vi "crio_FPGA_VCA_Force_Sine_Sweep.vi"() -> ()   [LabVIEW 2019]
uses:
  <vilib>/LabVIEW Targets/FPGA/cRIO/shared/nicrio_ModuleControls/nicrio_cRIO-9237_ExcitationVoltageRing.ctl
  <vilib>/LabVIEW Targets/FPGA/cRIO/shared/nicrio_ModuleControls/nicrio_cRIO-9237_DataRatesRing.ctl
  <vilib>/Platform/TimedLoop/XDataNode/timing_clust.ctl
  <vilib>/Platform/TimedLoop/XDataNode/nitl_modes.ctl
  <vilib>/Platform/TimedLoop/XDataNode/wakeup.ctl
  <vilib>/rvi/FXPMathLib/basic elements/FxpIntAccumulator/subVIs/nifxpmath_IntAccumulator_SimConfig.ctl
  <vilib>/rvi/FXPMathLib/FxpRectToPolar/subVIs/nifxpmath_RectToPolar_SimConfig.ctl
  <vilib>/rvi/Emulation/niFpgaSctlEmulationGetInTimedLoop.vi
  <vilib>/rvi/Emulation/niFpgaProcessEmulError.vi
  <vilib>/rvi/eio/common/nirviEmuTemplateMethod_errors.vi
  <vilib>/rvi/eio/common/nirviEmuTemplatePropertySet_errors.vi
  <vilib>/rvi/Emulation/niFpgaGetClockAttributes.vi
  <vilib>/rvi/Emulation/niFpgaEmulationReportErrorSimple.vi
  <vilib>/rvi/Emulation/niFpgaCriticalErrorInLSC.vi
  <vilib>/rvi/Analysis/common/codeGenErrors/XNode/niFpgaXNodeCodeGenErrorHandle.vi
  <vilib>/rvi/FXPMathLib/basic elements/FxpIntAccumulator/simVIs/DllFxpIntAccumulator_sub.vi
  <vilib>/rvi/FXPMathLib/FxpRectToPolar/simVIs/DllFxpRectToPolarTemp_sub.vi
  <vilib>/eio/EIOMethodNode/EIOMethodNode.xnode
  <vilib>/eio/EIOPropertyNode/EIOPropertyNode.xnode
  <vilib>/eio/EIONode/EIONode.xnode
  <vilib>/rvi/FXPMathLib/FxpInterpret/XNode/nifxpmath_Interpret.xnode
  <vilib>/rvi/FXPMathLib/FxpMul/XNode/nifxpmath_Multiplier.xnode
  <vilib>/rvi/FXPMathLib/FxpAdd/XNode/nifxpmath_Add.xnode
  <vilib>/rvi/Analysis/measure/mean-var-std/XNode/niFpgaMean-Var-Std.xnode
  <vilib>/platform/TimedLoop/XDataNode/XDataNode.xnode
  <vilib>/rvi/FXPMathLib/basic elements/FxpIntAccumulator/XNode/nifxpmath_IntAccumulator.xnode
  <vilib>/rvi/FXPMathLib/FxpRectToPolar/XNode/nifxpmath_RectToPolar.xnode
  <vilib>/rvi/FXPMathLib/sim/FxpSim.dll
  <vilib>/Platform/TimedLoop/XDataNode/XDNodeRunTimeDep.lvlib
  <vilib>/rvi/eio/common/nirviEmuTemplatePropertyGet_errors.vi
  <vilib>/rvi/eio/common/nirviEmuTemplatePropertyGet_noerrors.vi
  <vilib>/rvi/eio/common/nirviEmuTemplatePropertySet_noerrors.vi
panel:
  out "scaled load cell reading":fxp<+/-,24,24>
  out "error out":errorcluster {"code" format="%.0x"}
  in  "Data Rate":T1=1 items=["50.000 kS/s (NI 9237)"=1, "25.000 kS/s (NI 9237)"=2, "16.667 kS/s (NI 9237)"=3, "12.500 kS/s (NI 9237)"=4, "10.000 kS/s (NI 9237)"=5, "8.333 kS/s (NI 9237)"=6, "7.143 kS/s (NI 9237)"=7, "6.250 kS/s (NI 9237)"=8, "5.556 kS/s (NI 9237)"=9, "5.000 kS/s (NI 9237)"=10, "4.545 kS/s (NI 9237)"=11, "4.167 kS/s (NI 9237)"=12, "3.846 kS/s (NI 9237)"=13, "3.571 kS/s (NI 9237)"=14, "3.333 kS/s (NI 9237)"=15, "3.125 kS/s (NI 9237)"=16, "2.941 kS/s (NI 9237)"=17, "2.778 kS/s (NI 9237)"=18, "2.632 kS/s (NI 9237)"=19, "2.500 kS/s (NI 9237)"=20, "2.381 kS/s (NI 9237)"=21, "2.273 kS/s (NI 9237)"=22, "2.174 kS/s (NI 9237)"=23, "2.083 kS/s (NI 9237)"=24, "2.000 kS/s (NI 9237)"=25, "1.923 kS/s (NI 9237)"=26, "1.852 kS/s (NI 9237)"=27, "1.786 kS/s (NI 9237)"=28, "1.724 kS/s (NI 9237)"=29, "1.667 kS/s (NI 9237)"=30, "1.613 kS/s (NI 9237)"=31]
  in  "Excitation Voltage":T2 items=["2.5 Volts", "3.3 Volts", "5.0 Volts", "10.0 Volts", "External Excitation"]
  in  "Half-Bridge Enable":bool
  in  "Finite?":bool=TRUE
  in  "Samples per Channel":u32=1000
  out "Mod1/AI0":fxp<+/-,24,-4>
  in  "Loop Rate (uSec)":u32
  in  "Shunt Cal Enable":bool
  in  "sweep frequency (periods/tick)":fxp<+,32,0>=1.25030055642128e-06
  out "sine out":i16
  out "sin_fxp":fxp<+/-,16,1>
  out "cos_fxp":fxp<+/-,16,1>
  out "cosine out":i16
  in  "Lock_loop_rate":u32 caption="Count(uSec)"
  in  "Lock_debug":bool
  out "magnitude":fxp<+,32,6>
  out "phase (pi)":fxp<+/-,16,2>
  out "output valid":bool
  out "sin*input":fxp<+/-,32,6>
  out "cos*input":fxp<+/-,32,6>
  out "lock_input":fxp<+/-,24,24>
  in  "sin_gain":fxp<+,32,1>=0.5
  in  "sin_offset":fxp<+/-,16,3>=0.5
  out "ControllerPWM Output":sgl
  in  "stop":bool
  in  "DC PWM Period (microsec)":i16=50
  # "1Hz -> sweep frequency: 2.5e-8\n5H -> 1.25e-7"
  # "DRV8256 Specs:\n\n0 0: Brake Low\n1 1: Brake High\nPWM 0\n0 PWM"
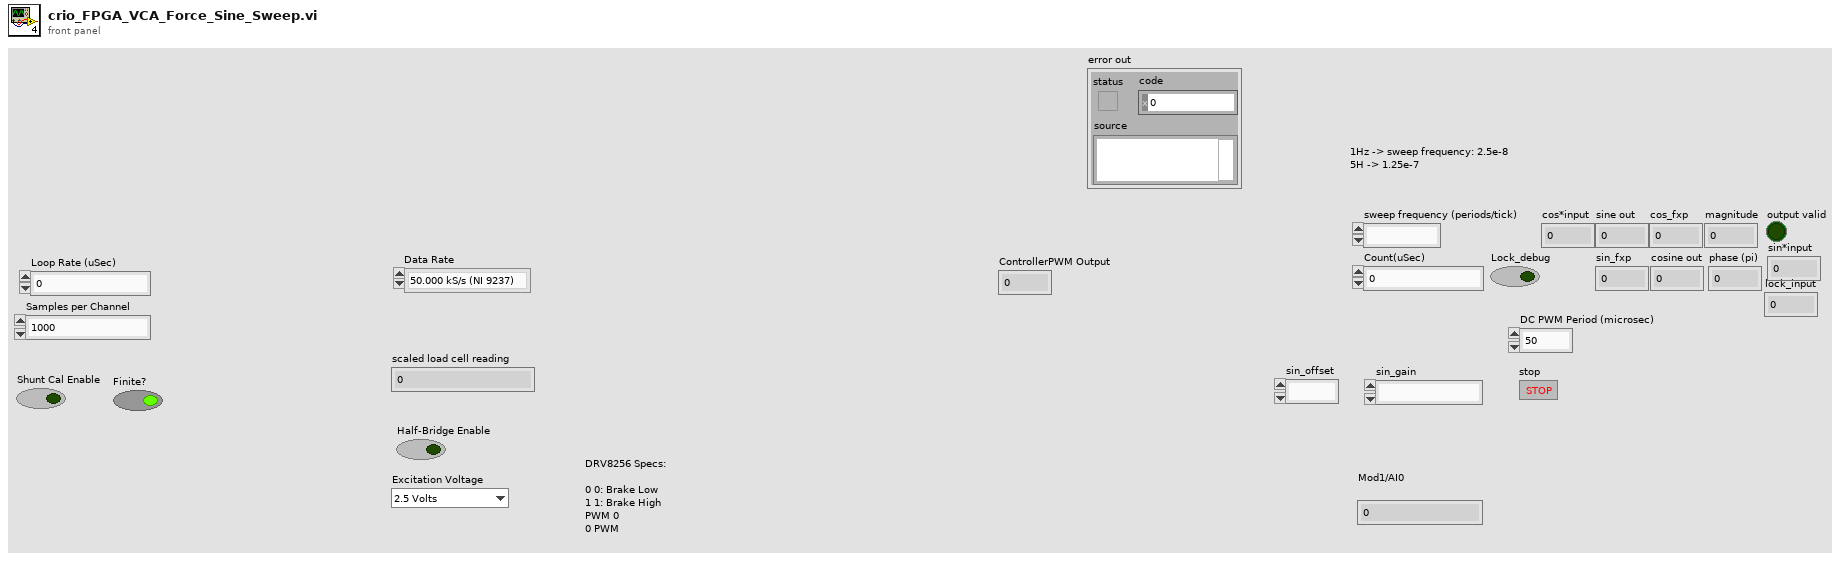
[diagram p1: front panel]
types:
  T1 = typedef "nicrio_cRIO-9237_DataRatesRing.ctl" = u8
  T2 = typedef "nicrio_cRIO-9237_ExcitationVoltageRing.ctl" = u8
  T3 = typedef "XDNodeRunTimeDep.lvlib/timing_clust.ctl" = cluster{"Expected End [f-1]":u64, "Actual End [f-1]":u64, "Finished Late? [f-1]":bool, "Expected End [i-1]":u64, "Actual End [i-1]":u64, "Finished Late? [i-1]":bool, "Expected Start [i]":u64, "Actual Start [i]":u64, "Expected Start [f]":u64, "Actual Start [f]":u64, "Source Name":string, "Structure Name":string, "Period":i64, "Deadline":i64, "Offset":i64, "Start":i64, "Priority":i32, "Timeout":i32, "Mode":T4, "Wakeup Reason":T5, "Error":errorcluster, "Source Type":string, "Secondary Source Type":string, "Global End Time":u64, "Global Start Time":u64, "Frame Duration":u64, "Iteration Duration":u64, "Assigned CPU":i32, "I/O Scan Engine Mode":u32}
  T4 = typedef "XDNodeRunTimeDep.lvlib/nitl_modes.ctl" = enum32{"No Change", "Process missed periods, maintain original phase", "Discard missed periods, maintain original phase", "Process missed periods, ignore original phase", "Discard missed periods, ignore original phase"}
  T5 = typedef "XDNodeRunTimeDep.lvlib/wakeup.ctl" = enum32{"Normal", "Aborted", "Asynchronous wakeup", "Timing source error", "Timed loop error", "Timeout"}
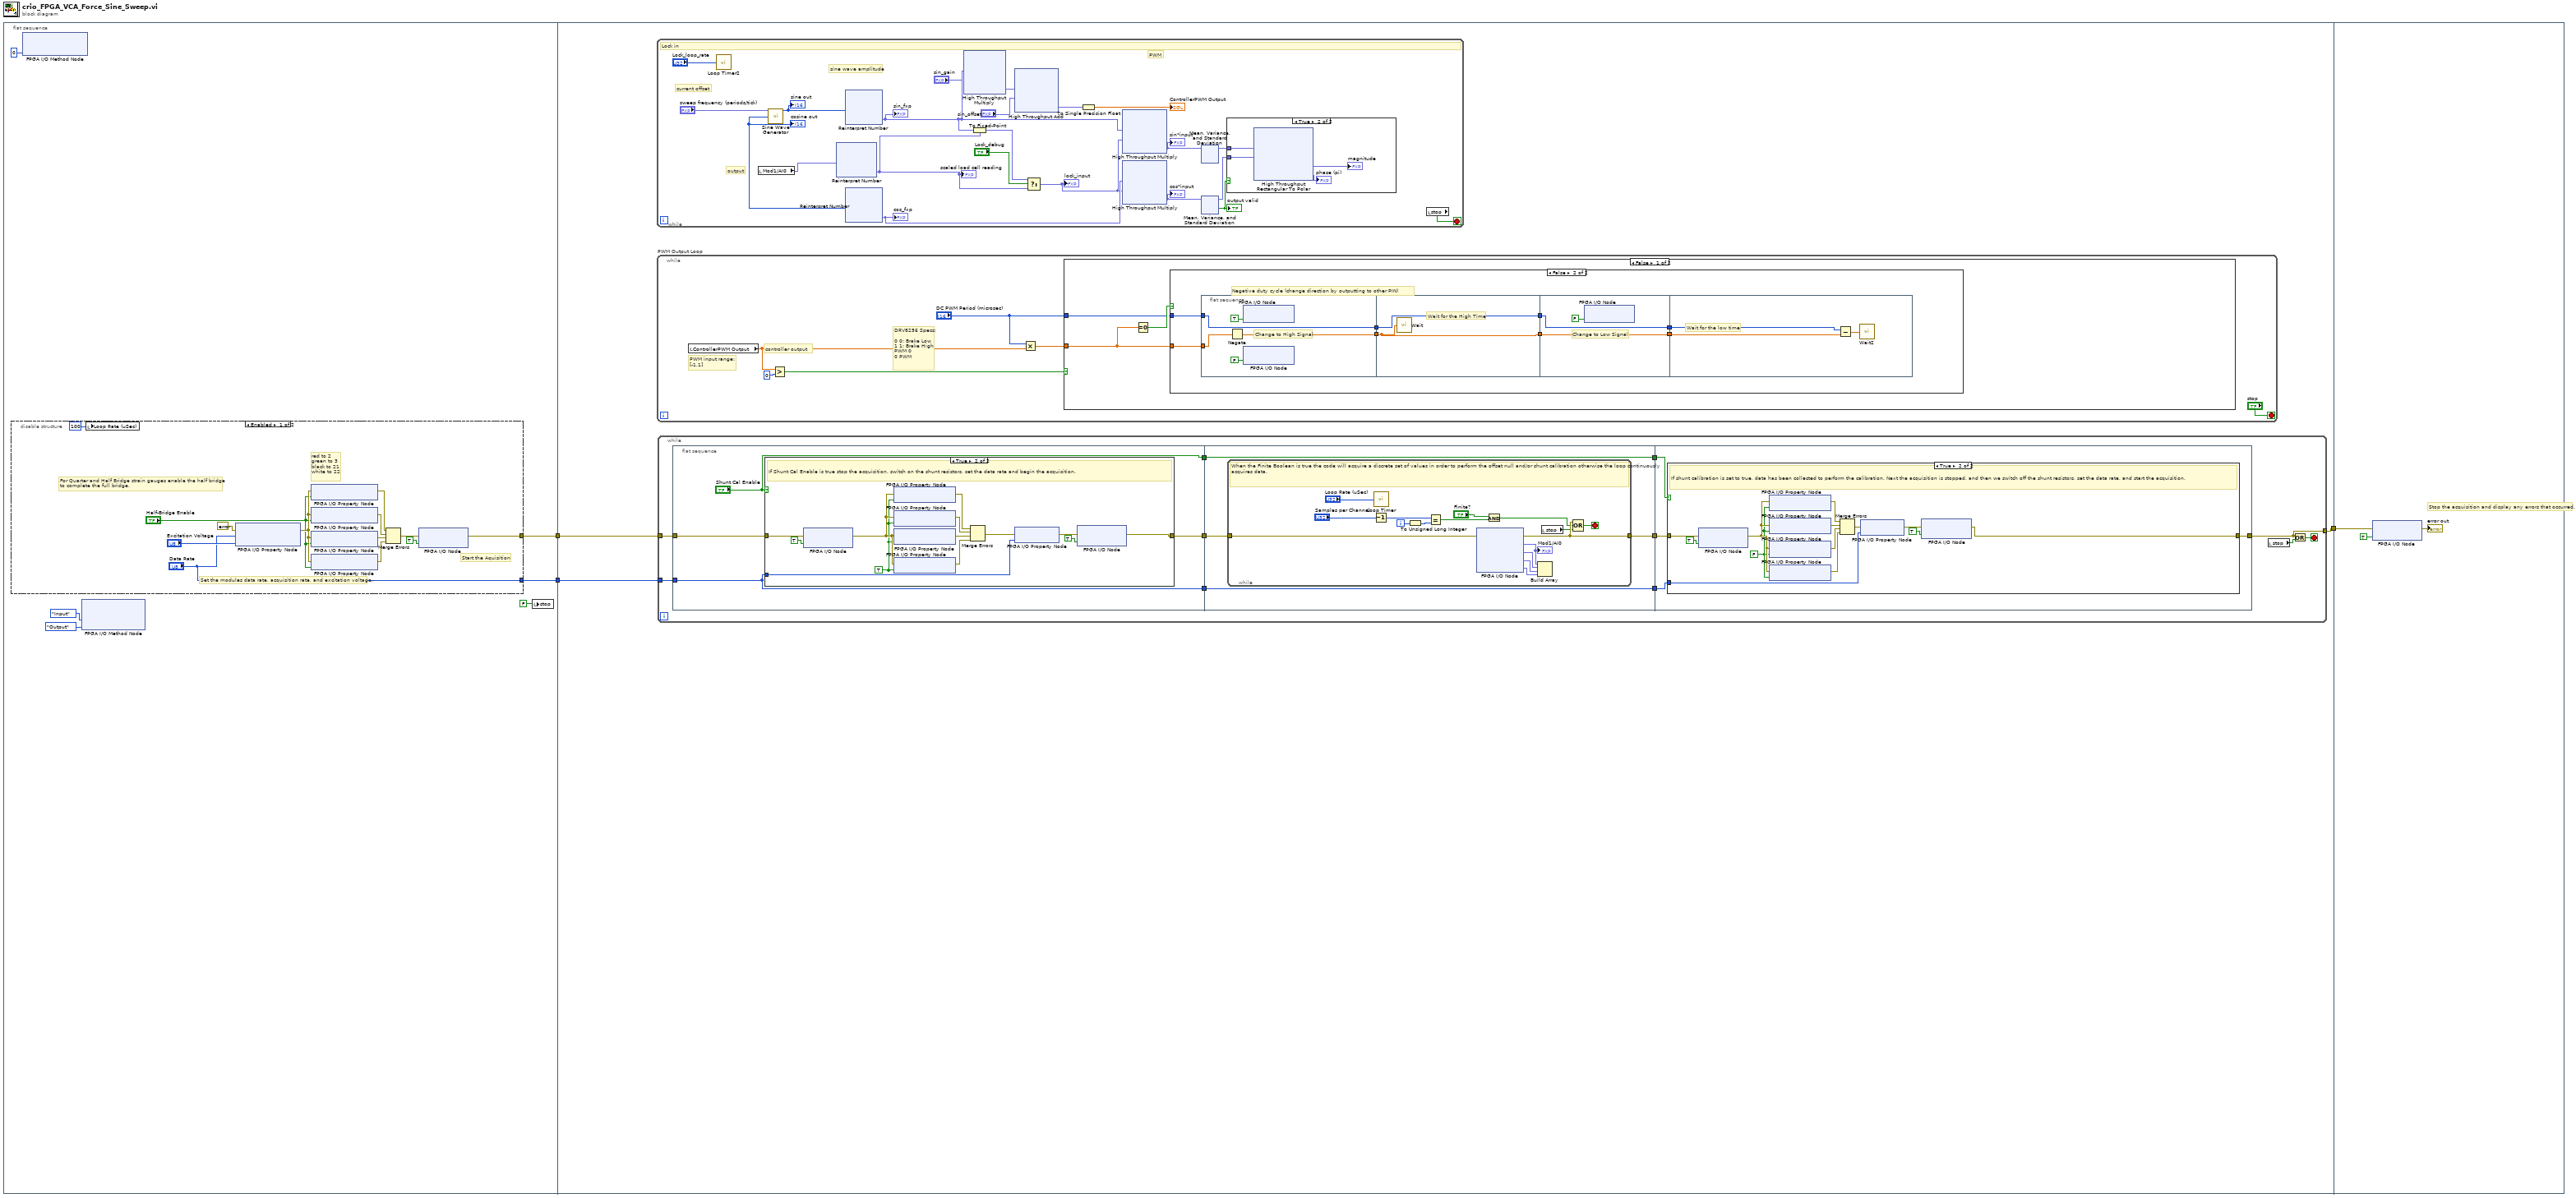
[diagram p0: block diagram]
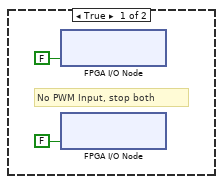
[diagram p6: hidden frame]
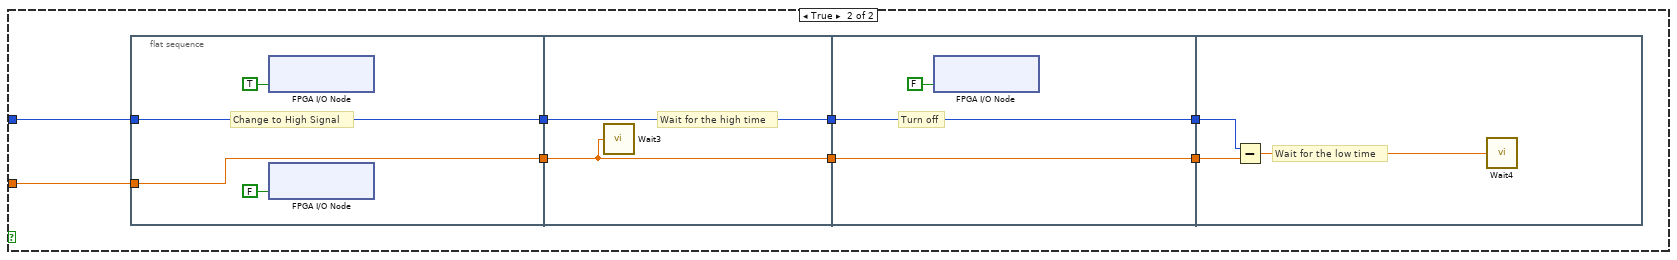
[diagram p7: hidden frame]
diagram:
  n1 = flat-sequence {
    tunnel: [w5] -> w3
    tunnel: [w4] -> w2
    tunnel: w3 -> [w25]
    tunnel: w2 -> [w24]
    tunnel: [w23] -> w1
    tunnel: w1 -> [w360]
    frame #0 {
      n2 = disable-structure shown="Enabled" {
        disable-tunnel: ["Data Rate" _] -> w5
        disable-tunnel: [w10 _] -> w4
        frame Enabled {
          # "red to 2\ngreen to 3\nblack to 21\nwhite to 22"
          # "Start the Aquisition"
          # "For Quarter and Half Bridge strain gauges enable the half bridge \nto complete the full bridge."
          # "Set the modules data rate, acquisition rate, and excitation voltage."
          n3 = local write "Loop Rate (uSec)"(u32 100 ("Loop Rate (uSec)")) -> ()
          n4 = xnode "FPGA I/O Property Node"("error in"=errorcluster {"status"=FALSE, "code"=0, "source"=""}, "Data Rate"="Data Rate", "Excitation Voltage"="Excitation Voltage") -> ("error out"=w20:errorcluster)  [unwired: 1 in, 1 out]
          n5 = xnode "FPGA I/O Property Node"("error in"=w20, "Half-Bridge Enable"="Half-Bridge Enable") -> ("error out"=w16:errorcluster)  [unwired: 1 in, 1 out]
          n6 = xnode "FPGA I/O Property Node"("error in"=w20, "Half-Bridge Enable"="Half-Bridge Enable") -> ("error out"=w17:errorcluster)  [unwired: 1 in, 1 out]
          n7 = xnode "FPGA I/O Property Node"("error in"=w20, "Half-Bridge Enable"="Half-Bridge Enable") -> ("error out"=w18:errorcluster)  [unwired: 1 in, 1 out]
          n8 = xnode "FPGA I/O Property Node"("error in"=w20, "Half-Bridge Enable"="Half-Bridge Enable") -> ("error out"=w19:errorcluster)  [unwired: 1 in, 1 out]
          n9 = Merge Errors(w16, w17, w18, w19) -> (w21:errorcluster)
          n10 = xnode "FPGA I/O Node"("error in"=w21, "Mod6/Start"=TRUE ("Mod1/Stop")) -> ("error out"=w10:errorcluster)  [unwired: 1 in, 1 out]
        }
        frame Disabled {
        }
      }
      n11 = xnode "FPGA I/O Method Node"("Enable"=u8 0) -> ()  [unwired: 1 in, 1 out]
      n12 = xnode "FPGA I/O Method Node"("DIO 7:4"=enum8{"No Change", "Input", "Output"}."Input", "DIO 3:0"=enum8{"No Change", "Input", "Output"}."Output") -> ()  [unwired: 1 in, 1 out]
      n13 = local write "stop"(FALSE ("stop")) -> ()
    }
    frame #1 {
      n14 = while {
        stop <- w95 stop-if-true
        # "output"
        # "PWM"
        # "current offset"
        # "sine wave amplitude"
        # "Lock in"
        n15 = call "Loop Timer2"("Count(uSec)"="Lock_loop_rate") -> ()  [unwired: 1 out]
        n16 = local read "Mod1/AI0"() -> (w94:fxp<+/-,24,-4>)
        n17 = call "Sine Wave Generator"("frequency (periods/tick)"="sweep frequency (periods/tick)") -> ("sine out"=w113:i16, "cosine out"=w112:i16)  [unwired: 13 in]
        "sine out" <- w113
        "cosine out" <- w112
        n18 = xnode "Reinterpret Number"("x"=w94) -> ("y"=w93:fxp<+/-,24,16>)
        "scaled load cell reading" <- w93
        n19 = xnode "Reinterpret Number"("x"=w113) -> ("y"=w101:fxp<+/-,16,1>)
        "sin_fxp" <- w101
        n20 = xnode "Reinterpret Number"("x"=w112) -> ("y"=w111:fxp<+/-,16,1>)
        "cos_fxp" <- w111
        n21 = xnode ("High Throughput Multiply")("x"=w101, "y"="sin_gain") -> ("x*y"=w99:fxp<+/-,48,2>)
        n22 = To Fixed-Point(fixed-point type=w93, number=w101) -> (fixed-point=w108:fxp<+/-,24,16>)
        n23 = xnode ("High Throughput Add")("x"=w99, "y"="sin_offset") -> ("x+y"=w97:fxp<+/-,50,4>)
        n24 = Select(t=w108, s="Lock_debug", f=w93) -> (s? t:f=w102:fxp<+/-,24,16>)
        "lock_input" <- w102
        n25 = To Single Precision Float(number=w97) -> (single precision float=→"ControllerPWM Output":sgl)
        n26 = xnode ("High Throughput Multiply")("x"=w101, "y"=w102) -> ("x*y"=w106:fxp<+/-,40,17>)
        "sin*input" <- w106
        n27 = xnode ("High Throughput Multiply")("x"=w111, "y"=w102) -> ("x*y"=w107:fxp<+/-,40,17>)
        "cos*input" <- w107
        n28 = xnode "Mean, Variance, and Standard Deviation"("input data"=w106) -> ("mean"=w105:fxp<+/-,32,17>)  [unwired: 1 in, 1 out]
        n29 = xnode "Mean, Variance, and Standard Deviation"("input data"=w107) -> ("mean"=w104:fxp<+/-,32,17>, "output valid"=w103:bool)  [unwired: 1 in]
        "output valid" <- w103
        n30 = case shown="True" w103 {
          tunnel: w105 -> [_ w116]
          tunnel: w104 -> [_ w115]
          frame False {
          }
          frame True {
            n31 = xnode "High Throughput Rectangular To Polar"("x"=w116, "y"=w115) -> ("magnitude"=→"magnitude":fxp<+,32,17>, "phase (pi)"=→"phase (pi)":fxp<+/-,16,2>)
          }
        }
        n32 = local read "stop"() -> (w95:bool)
      }
      n33 = while "PWM Output Loop" {
        stop <- "stop" stop-if-true
        # "PWM input range:\n[-1,1]"
        # "DRV8256 Specs:\n\n0 0: Brake Low\n1 1: Brake High\nPWM 0\n0 PWM"
        # "controller output"
        n34 = local read "ControllerPWM Output"() -> (w308:sgl)
        n35 = Greater?(x=w308, y=i16 0) -> (0:w311:bool)
        n36 = Multiply(x="DC PWM Period (microsec)", y=w308) -> (x*y=w310:sgl)
        n37 = case shown="False" w311 {
          tunnel: w310 -> [w316 w347]
          tunnel: "DC PWM Period (microsec)" -> [w314 w346]
          frame False {
            n38 = Equal To 0?(x=w316) -> (x = 0?=w315:bool)
            n39 = case shown="False" w315 {
              tunnel: w316 -> [_ w326]
              tunnel: w314 -> [_ w319]
              frame True {
                # "No PWM Input, stop both"
                n40 = xnode "FPGA I/O Node"("Mod1/DIO1"=FALSE) -> ()  [unwired: 1 in, 1 out]
                n41 = xnode "FPGA I/O Node"("Mod1/DIO0"=FALSE) -> ()  [unwired: 1 in, 1 out]
              }
              frame False {
                # "Negative duty cycle (change direction by outputting to other PIN)"
                n42 = flat-sequence {
                  tunnel: w326 -> [w329]
                  tunnel: [w328] -> w325
                  tunnel: [w327] -> w320
                  tunnel: w319 -> [w327]
                  tunnel: w325 -> [w333]
                  tunnel: [w333] -> w324
                  tunnel: [w332] -> w321
                  tunnel: w320 -> [w332]
                  tunnel: w324 -> [w335]
                  tunnel: [w335] -> w323
                  tunnel: [w334] -> w322
                  tunnel: w321 -> [w334]
                  tunnel: w323 -> [w339]
                  tunnel: w322 -> [w338]
                  frame #0 {
                    # "Change to High Signal"
                    n43 = Negate(x=w329) -> (-x=w328:sgl)
                    n44 = xnode "FPGA I/O Node"("Mod1/DIO1"=TRUE) -> ()  [unwired: 1 in, 1 out]
                    n45 = xnode "FPGA I/O Node"("Mod1/DIO0"=FALSE) -> ()  [unwired: 1 in, 1 out]
                  }
                  frame #1 {
                    # "Wait for the High Time"
                    n46 = call "Wait"("Count(uSec)"=w333) -> ()  [unwired: 1 out]
                  }
                  frame #2 {
                    # "Change to Low Signal"
                    n47 = xnode "FPGA I/O Node"("Mod1/DIO1"=FALSE) -> ()  [unwired: 1 in, 1 out]
                  }
                  frame #3 {
                    # "Wait for the low time"
                    n48 = Subtract(x=w338, y=w339) -> (x-y=w337:sgl)
                    n49 = call "Wait2"("Count(uSec)"=w337) -> ()  [unwired: 1 out]
                  }
                }
              }
            }
          }
          frame True {
            n50 = flat-sequence {
              tunnel: w347 -> [w348]
              tunnel: w346 -> [w349]
              tunnel: [w349] -> w343
              tunnel: [w348] -> w342
              tunnel: [w353] -> w344
              tunnel: w343 -> [w353]
              tunnel: w342 -> [w352]
              tunnel: [w352] -> w341
              tunnel: [w355] -> w345
              tunnel: w344 -> [w355]
              tunnel: w341 -> [w354]
              tunnel: [w354] -> w340
              tunnel: w345 -> [w359]
              tunnel: w340 -> [w357]
              frame #0 {
                # "Change to High Signal"
                n51 = xnode "FPGA I/O Node"("Mod1/DIO0"=TRUE) -> ()  [unwired: 1 in, 1 out]
                n52 = xnode "FPGA I/O Node"("Mod1/DIO1"=FALSE ("ConnectorB/DIO9")) -> ()  [unwired: 1 in, 1 out]
              }
              frame #1 {
                # "Wait for the high time"
                n53 = call "Wait3"("Count(uSec)"=w352) -> ()  [unwired: 1 out]
              }
              frame #2 {
                # "Turn off"
                n54 = xnode "FPGA I/O Node"("Mod1/DIO0"=FALSE) -> ()  [unwired: 1 in, 1 out]
              }
              frame #3 {
                # "Wait for the low time"
                n55 = Subtract(x=w359, y=w357) -> (x-y=w358:sgl)
                n56 = call "Wait4"("Count(uSec)"=w358) -> ()  [unwired: 1 out]
              }
            }
          }
        }
      }
      n57 = while {
        tunnel: w24 -> [w36]
        tunnel: [w33] -> w23
        tunnel: w25 -> [w31]
        stop <- w34 stop-if-true
        n58 = flat-sequence {
          tunnel: [w39] -> w32
          tunnel: [w38] -> w29
          tunnel: ["Shunt Cal Enable"] -> w28
          tunnel: w31 -> [w38]
          tunnel: w36 -> [w40]
          tunnel: [w57] -> w35
          tunnel: w32 -> [w58]
          tunnel: [w56] -> w30
          tunnel: w29 -> [w56]
          tunnel: w28 -> [w55]
          tunnel: [w55] -> w27
          tunnel: [w77] -> w33
          tunnel: w35 -> [w78]
          tunnel: w30 -> [w75]
          tunnel: w27 -> [w76]
          frame #0 {
            n59 = case shown="True" "Shunt Cal Enable" {
              tunnel: w40 -> [w41 w51]
              tunnel: [w41 w49] -> w39
              tunnel: w38 -> [_ w46]
              frame False {
              }
              frame True {
                w44 = TRUE ("Shunt Cal Enable")
                # "If Shunt Cal Enable is true stop the acquisition, switch on the shunt resistors, set the data rate and begin the acquisition."
                n60 = xnode "FPGA I/O Node"("error in"=w51, "Mod6/Stop"=TRUE ("Mod1/Stop")) -> ("error out"=w50:errorcluster)  [unwired: 1 in, 1 out]
                n61 = xnode "FPGA I/O Property Node"("error in"=w50, "Shunt Cal Enable"=w44) -> ("error out"=w54:errorcluster)  [unwired: 1 in, 1 out]
                n62 = xnode "FPGA I/O Property Node"("error in"=w50, "Shunt Cal Enable"=w44) -> ("error out"=w42:errorcluster)  [unwired: 1 in, 1 out]
                n63 = xnode "FPGA I/O Property Node"("error in"=w50, "Shunt Cal Enable"=w44) -> ("error out"=w53:errorcluster)  [unwired: 1 in, 1 out]
                n64 = xnode "FPGA I/O Property Node"("error in"=w50, "Shunt Cal Enable"=w44) -> ("error out"=w52:errorcluster)  [unwired: 1 in, 1 out]
                n65 = Merge Errors(w54, w42, w53, w52) -> (w47:errorcluster)
                n66 = xnode "FPGA I/O Property Node"("error in"=w47, "Data Rate"=w46) -> ("error out"=w48:errorcluster)  [unwired: 1 in, 1 out]
                n67 = xnode "FPGA I/O Node"("error in"=w48, "Mod6/Start"=TRUE ("Mod1/Start")) -> ("error out"=w49:errorcluster)  [unwired: 1 in, 1 out]
              }
            }
          }
          frame #1 {
            n68 = while {
              tunnel: w58 -> [w60]
              tunnel: [w64] -> w57
              i -> [w68]
              stop <- w61 stop-if-true
              # "When the Finite Boolean is true the code will acquire a discrete set of values in order to perform the offset null and/or shunt calibration otherwise the loop continuously acquires data."
              n69 = Decrement(x="Samples per Channel") -> (x-1=w70:u32)
              n70 = call "Loop Timer"("Count(uSec)"="Loop Rate (uSec)") -> ()  [unwired: 1 out]
              n71 = To Unsigned Long Integer(number=w68) -> (unsigned 32bit integer=w69:u32)
              n72 = Equal?(x=w70, y=w69) -> (x = y?=w65:bool)
              n73 = xnode "FPGA I/O Node"("error in"=w60) -> ("error out"=w64:errorcluster, "Mod6/AI0"=w74:fxp<+/-,24,-4>, "Mod6/AI1"=w73:fxp<+/-,24,-4>, "Mod6/AI2"=w71:fxp<+/-,24,-4>, "Mod6/AI3"=w72:fxp<+/-,24,-4>)  [unwired: 4 in, 4 out]
              "Mod1/AI0" <- w74
              n74 = And(x="Finite?", y=w65) -> (x .and. y?=w63:bool)
              n75 = Build Array(w74, w73, w71, w72) -> ()  [unwired: 1 out]
              n76 = local read "stop"() -> (w62:bool)
              n77 = Compound Arithmetic op=OR(w64, w63, w62) -> (w61:bool)
            }
          }
          frame #2 {
            n78 = case shown="True" w76 {
              tunnel: w78 -> [w79 w88]
              tunnel: [w79 w86] -> w77
              tunnel: w75 -> [_ w83]
              frame False {
              }
              frame True {
                w82 = FALSE ("Shunt Cal Enable")
                # "If shunt calibration is set to true, data has been collected to perform the calibration. Next the acquisition is stopped, and then we switch off the shunt resistors, set the data rate, and start the acquisition."
                n79 = xnode "FPGA I/O Node"("error in"=w88, "Mod6/Stop"=TRUE ("Mod1/Stop")) -> ("error out"=w87:errorcluster)  [unwired: 1 in, 1 out]
                n80 = xnode "FPGA I/O Property Node"("error in"=w87, "Shunt Cal Enable"=w82) -> ("error out"=w92:errorcluster)  [unwired: 1 in, 1 out]
                n81 = xnode "FPGA I/O Property Node"("error in"=w87, "Shunt Cal Enable"=w82) -> ("error out"=w91:errorcluster)  [unwired: 1 in, 1 out]
                n82 = xnode "FPGA I/O Property Node"("error in"=w87, "Shunt Cal Enable"=w82) -> ("error out"=w90:errorcluster)  [unwired: 1 in, 1 out]
                n83 = xnode "FPGA I/O Property Node"("error in"=w87, "Shunt Cal Enable"=w82) -> ("error out"=w89:errorcluster)  [unwired: 1 in, 1 out]
                n84 = Merge Errors(w92, w91, w90, w89) -> (w84:errorcluster)
                n85 = xnode "FPGA I/O Property Node"("error in"=w84, "Data Rate"=w83) -> ("error out"=w85:errorcluster)  [unwired: 1 in, 1 out]
                n86 = xnode "FPGA I/O Node"("error in"=w85, "Mod6/Start"=TRUE ("Mod1/Start")) -> ("error out"=w86:errorcluster)  [unwired: 1 in, 1 out]
              }
            }
          }
        }
        n87 = local read "stop"() -> (w26:bool)
        n88 = Or(x=w33, y=w26) -> (x .or. y?=w34:bool)
      }
    }
    frame #2 {
      # "Stop the acquisition and display any errors that occurred."
      n89 = xnode "FPGA I/O Node"("error in"=w360, "Mod6/Stop"=TRUE ("Mod1/Stop")) -> ("error out"=→"error out":errorcluster)  [unwired: 1 in, 1 out]
    }
  }
